vi "Add Message Section.vi"(8 "error in":errorcluster, 10 "message name":string, 11 "bus controller in":T1 format="%.0x") -> (0 "error out":errorcluster, 2 "message":T1 format="%.0x", 3 "bus controller out":T1 format="%.0x")   [LabVIEW 2020, in "Ballard MIL-STD-1553 Scripting.lvlib"]
uses:
  Ballard MIL-STD-1553 Scripting.lvlib
  <vilib>/NI VeriStand/Custom Device API/Custom Device Item Ref.ctl
  Constants.vi
  <vilib>/NI VeriStand/Custom Device API/Custom Device API.lvlib
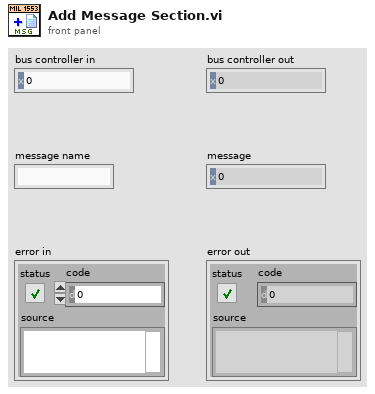
[diagram p1: front panel]
types:
  T1 = typedef "Custom Device API.lvlib/Custom Device Item Ref.ctl" = u64
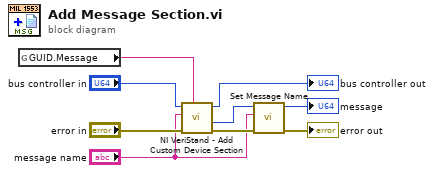
[diagram p0: block diagram]
diagram:
  n1 = global read "Constants.vi" "GUID.Message"() -> (w9:string)
  n2 = call <vilib>:"NI VeriStand - Add Custom Device Section.vi"("GUID (Default Section)"=w9, "error in (no error)"="error in", "Section Name"="message name", "Parent Ref in"="bus controller in") -> ("error out"=w5:errorcluster, "Section Ptr"=w6:T1, "Parent Ref out"=→"bus controller out":T1)  [unwired: 4 in, 1 out]
  n3 = call "Set Message Name.vi"("error in"=w5, "message name"="message name", "message in"=w6) -> ("error out"=→"error out":errorcluster, "message out"=→"message":T1)  [unwired: 7 in]
